vi "task_booleanNotifier.vi"(8 "error in (no error)":errorcluster, 10 "taskChannel":refnum<class "ITaskChannel.lvclass">, 11 "ITask in":refnum<class "ITask.lvclass">) -> (0 "error out":errorcluster, 3 "ITask out":refnum<class "ITask.lvclass">)   [LabVIEW 2023]
uses:
  TLC_Daemon.lvlib
  ITask/ITask.lvclass
  ITaskChannel/ITaskChannel.lvclass
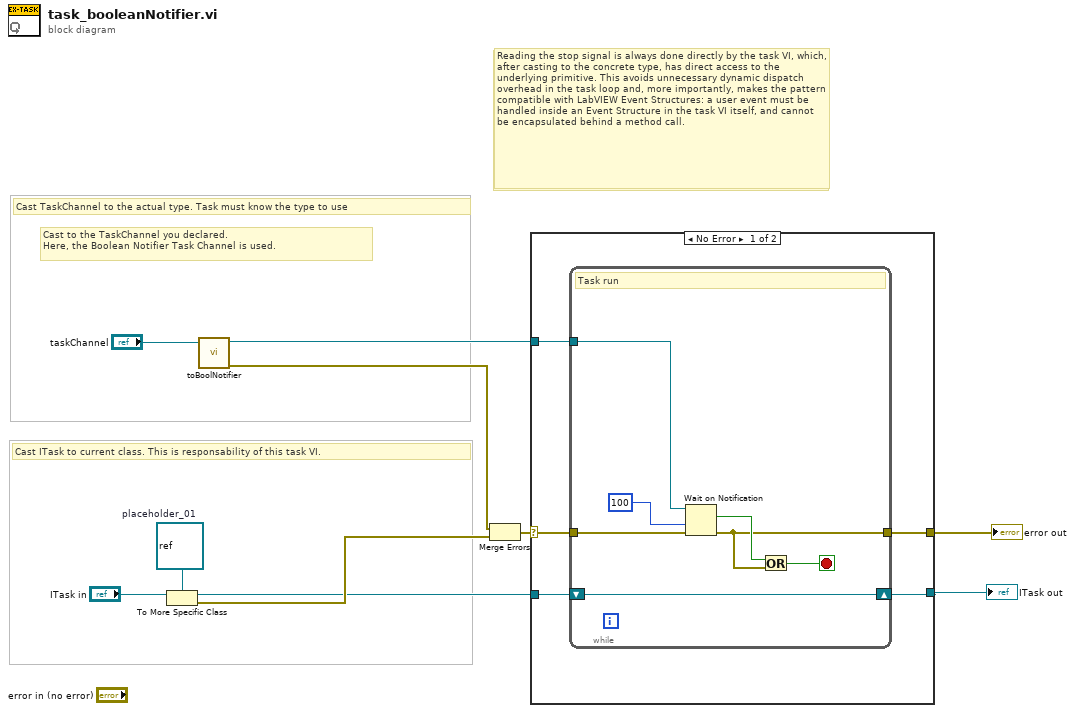
[diagram p0: block diagram]
diagram:
  w4 = refnum<class> refnum  # placeholder_01
  # "Cast to the TaskChannel you declared.\nHere, the Boolean Notifier Task Channel is used."
  # "The stop signal is always handled directly by the task VI, which, after casting to the concrete type, has direct access to the underlying primitive. This avoids unnecessary dynamic dispatch overhead in the task loop and, more importantly, makes the pattern compatible with LabVIEW Event Structures: a user event must be handled inside an Event Structure in the task VI itself, and cannot be encapsulated behind a method call."
  # "Reading the stop signal is always done directly by the task VI, which, after casting to the concrete type, has direct access to the underlying primitive. This avoids unnecessary dynamic dispatch overhead in the task loop and, more importantly, makes the pattern compatible with LabVIEW Event Structures: a user event must be handled inside an Event Structure in the task VI itself, and cannot be encapsulated behind a method call."
  # "Cast ITask to current class. This is responsability of this task VI."
  # "Cast TaskChannel to the actual type. Task must know the type to use"
  n1 = To More Specific Class(target class=w4, reference="ITask in") -> (specific class reference=w8:refnum<class>, error out=w9:errorcluster)  [unwired: 1 in]
  n2 = call "toBoolNotifier.vi"("ITaskChannel"="taskChannel") -> ("error out"=w1:errorcluster, "boolNotifier"=w2:refnum<notifier>)  [unwired: 9 in]
  n3 = Merge Errors(w1, w9) -> (w6:errorcluster)
  n4 = case shown="No Error" w6 {
    selector: w6 -> [w14 w24]
    tunnel: w2 -> [w15 _]
    tunnel: w8 -> [w11 w23]
    tunnel: [w12 w23] -> w7
    tunnel: [w13 w24] -> w5
    frame No Error {
      n5 = while {
        tunnel: w15 -> [w22]
        tunnel: w14 -> [w18]
        tunnel: [w17] -> w13
        shift-right: [w16] -> w12
        shift-left: w11 -> [w16]
        stop <- w19 stop-if-true
        # "Task run"
        n6 = Wait on Notification(notifier=w22, timeout in ms (-1)=100, error in (no error)=w18) -> (notification=w20:bool, error out=w17:errorcluster)  [unwired: 1 in, 2 out]
        n7 = Or(x=w20, y=w17) -> (x .or. y?=w19:bool)
      }
    }
    frame Error {
    }
  }
  "error out" <- w5
  "ITask out" <- w7
